vi "MIC communication_MD.vi"() -> ()   [LabVIEW 2012]
uses:
  <vilib>/Utility/VariantDataType/Type.ctl
  GFG/GFGstringGet.vi
  <vilib>/Instr/_visa.llb/VISA Configure Serial Port (Instr).vi
  GFG/GFG library.lvlib
  <vilib>/Utility/VariantDataType/VariantType.lvlib
panel:
  out "read buffer":string
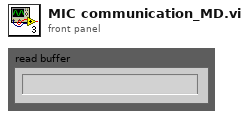
[diagram p1: front panel]
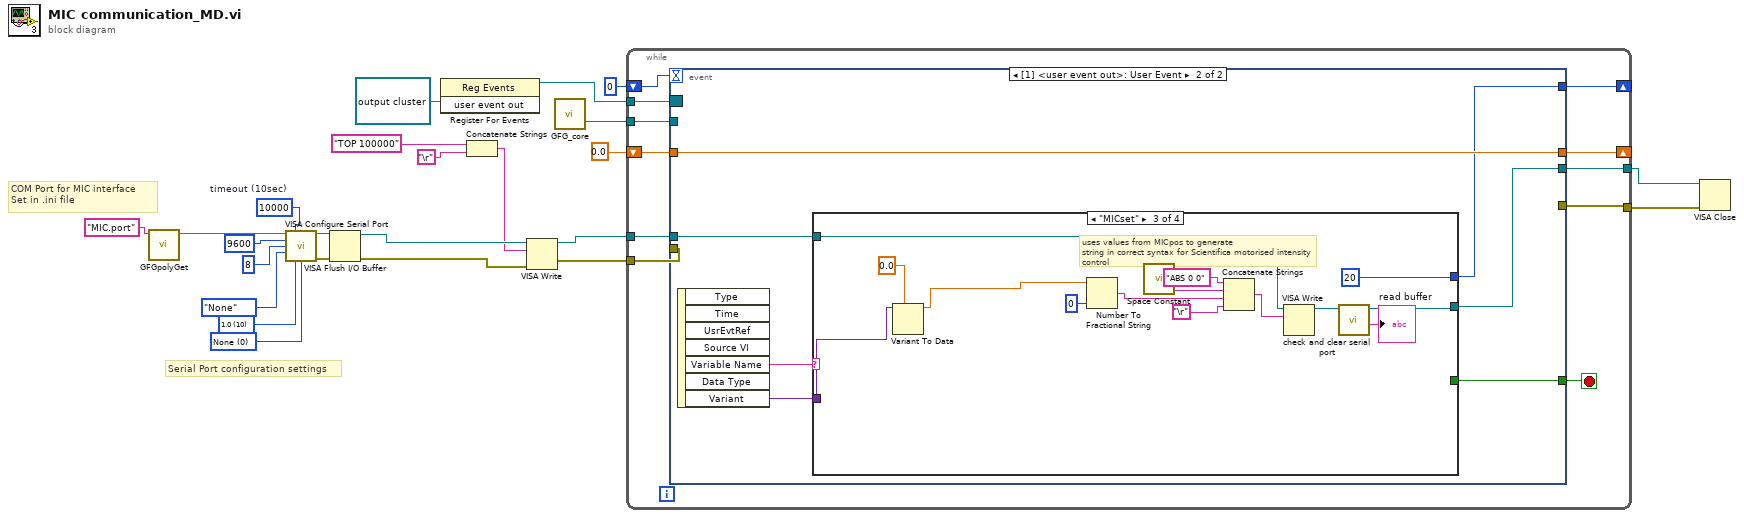
[diagram p0: block diagram]
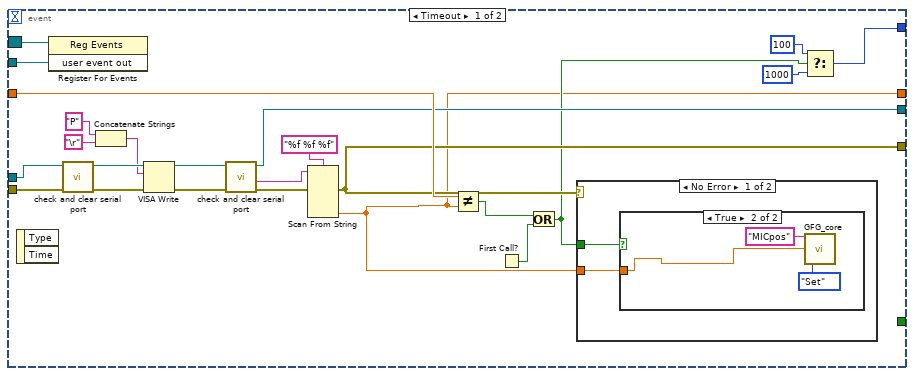
[diagram p2: hidden frame]
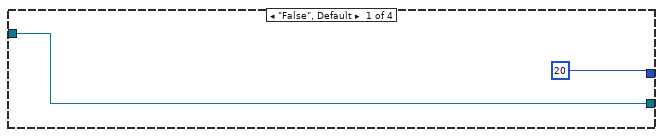
[diagram p5: hidden frame]
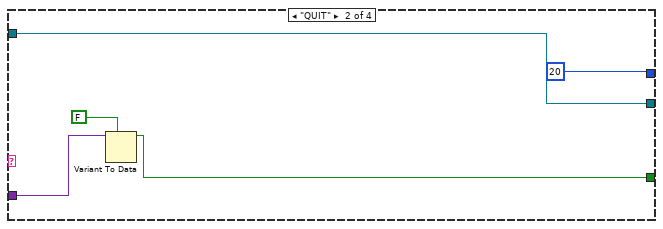
[diagram p6: hidden frame]
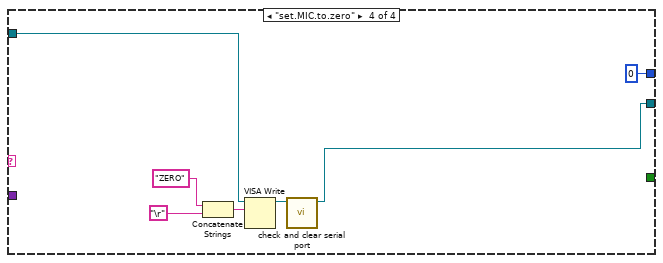
[diagram p7: hidden frame]
diagram:
  w18 = u16 0 items=["None", "XON/XOFF", "RTS/CTS", "XON/XOFF & RTS/CTS", "DTR/DSR", "XON/XOFF & DTR/DSR"] ("flow control (0:none)")
  w19 = u16 10 items=["1.0"=10, "1.5"=15, "2.0"=20] ("stop bits (10: 1 bit)")
  w23 = u32 10000  # timeout (10sec)
  # "COM Port for MIC interface\nSet in .ini file"
  # "Serial Port configuration settings"
  n1 = call-poly "GFGpolyGet.vi"("Variable Name in"="MIC.port") -> ("String"=w15:string)  [unwired: 10 in]
  n2 = call-poly "VISA Configure Serial Port"("VISA resource name"=w15, "timeout (10sec)"=w23, "baud rate (9600)"=u32 9600, "data bits (8)"=u16 8, "parity (0:none)"=enum16{"None", "Odd", "Even", "Mark", "Space"}."None", "stop bits (10: 1 bit)"=w19, "flow control (0:none)"=w18) -> ("VISA resource name out"=w17:refnum<visa-resource-name>, "error out"=w16:errorcluster)  [unwired: 7 in]
  n3 = VISA Flush I/O Buffer(VISA resource name=w17, error in (no error)=w16) -> (VISA resource name out=w7:refnum<visa-resource-name>, error out=w2:errorcluster)  [unwired: 1 in]
  n4 = register-events(refnum<user-event> refnum ("user event out")) -> (reference out=w9:refnum<event-registration>)  [unwired: 2 in, 1 out]
  n5 = Concatenate Strings("TOP 100000" ("write buffer"), "\r") -> (w4:string)
  n6 = VISA Write(VISA resource name=w7, write buffer=w4, error in (no error)=w2) -> (VISA resource name out=w3:refnum<visa-resource-name>, error out=w1:errorcluster)  [unwired: 1 out]
  n7 = call "GFG_core.vi"() -> ("user event out"=w13:refnum<user-event>)  [unwired: 13 in, 6 out]
  n8 = while {
    tunnel: [w35] -> w12
    tunnel: w3 -> [w34]
    shift-right: [w33] -> _
    shift-left: 0.0 -> [w31]
    tunnel: w1 -> [w30]
    tunnel: [w29] -> w11
    shift-right: [w27] -> _
    shift-left: 0 -> [w28]
    tunnel: w13 -> [w26]
    tunnel: w9 -> [w25]
    stop <- w32 stop-if-true
    n9 = event shown="[1] <user event out>: User Event" {
      selector: w25 -> [w39 _]
      dyn-events: _ -> [_ _]
      timeout: w28 -> [_ _]
      tunnel: [w47 w67] -> w35
      tunnel: w34 -> [w56 w68]
      tunnel: [w36 w66] -> w33
      tunnel: [_ w69] -> w32
      tunnel: w31 -> [w59 w66]
      tunnel: w30 -> [w54 _]
      tunnel: [w58 _] -> w29
      tunnel: [w42 w65] -> w27
      tunnel: w26 -> [w38 _]
      event Timeout {
        n10 = event-data() -> ()  [unwired: 1 in, 2 out]
        n11 = register-events(reference=w39, w38) -> ()  [unwired: 1 in, 2 out]
        n12 = call "check and clear serial port.vi"("error in (no error)"=w54, "VISA resource name in"=w56) -> ("error out"=w53:errorcluster, "VISA resource name out"=w55:refnum<visa-resource-name>)  [unwired: 6 in, 2 out]
        n13 = Concatenate Strings("P" ("write buffer"), "\r") -> (w45:string)
        n14 = VISA Write(VISA resource name=w55, write buffer=w45, error in (no error)=w53) -> (VISA resource name out=w49:refnum<visa-resource-name>, error out=w50:errorcluster)  [unwired: 1 out]
        n15 = call "check and clear serial port.vi"("error in (no error)"=w50, "VISA resource name in"=w49) -> ("error out"=w48:errorcluster, "read buffer"=w46:string, "VISA resource name out"=w47:refnum<visa-resource-name>)  [unwired: 6 in, 1 out]
        n16 = Scan From String(format string="%f %f %f", input string=w46, error in=w48) -> (error out=w58:errorcluster, output 3=w36:dbl)  [unwired: 6 in, 2 out]
        n17 = Not Equal?(x=w59, y=w36) -> (x != y?=w37:bool)
        n18 = First Call?() -> (First Call?: T/F=w41:bool)
        n19 = Or(x=w37, y=w41) -> (x .or. y?=w40:bool)
        n20 = case shown="No Error" w58 {
          tunnel: w36 -> [w61 _]
          tunnel: w40 -> [w60 _]
          frame No Error {
            n21 = case shown="True" w60 {
              tunnel: w61 -> [_ w62]
              frame False {
              }
              frame True {
                n22 = call "GFG_core.vi"("Variable Name in"="MICpos", "Variant in"=w62, "Action"=enum16{"Init", "Set", "Get"}."Set") -> ()  [unwired: 10 in, 7 out]
              }
            }
          }
          frame Error {
          }
        }
        n23 = Select(t=100, s=w40, f=1000) -> (s? t:f=w42:i32)
      }
      event User Event {
        n24 = event-data() -> ("Variable Name"=w71:string, "Variant"=w70:variant)  [unwired: 1 in, 5 out]
        n25 = case shown="\"MICset\"" w71 {
          tunnel: [_ w76 _ _] -> w69
          tunnel: w70 -> [_ w78 w84 _]
          tunnel: w68 -> [w73 w75 w89 w95]
          tunnel: [w73 w75 w87 w94] -> w67
          tunnel: [20 20 20 0] -> w65
          frame "False", Default {
          }
          frame "QUIT" {
            n26 = Variant To Data(type=FALSE ("NewVal"), Variant=w78) -> (data=w76:bool)  [unwired: 1 in, 1 out]
          }
          frame "MICset" {
            # "uses values from MICpos to generate\nstring in correct syntax for Scientifica motorised intensity control"
            n27 = Variant To Data(type=0.0 ("moveZabs"), Variant=w84) -> (data=w81:dbl)  [unwired: 1 in, 1 out]
            n28 = Number To Fractional String(number=w81, precision (6)=i16 0) -> (F-format string=w92:string)  [unwired: 2 in]
            n29 = call <vilib>:"Space Constant.vi"() -> ("String"=w91:string)
            n30 = Concatenate Strings("ABS 0 0" ("string"), w91, w92, "\r") -> (w86:string)
            n31 = VISA Write(VISA resource name=w89, write buffer=w86) -> (VISA resource name out=w88:refnum<visa-resource-name>)  [unwired: 1 in, 2 out]
            n32 = call "check and clear serial port.vi"("VISA resource name in"=w88) -> ("read buffer"=→"read buffer":string, "VISA resource name out"=w87:refnum<visa-resource-name>)  [unwired: 7 in, 2 out]
          }
          frame "set.MIC.to.zero" {
            n33 = Concatenate Strings("ZERO" ("write buffer"), "\r") -> (w96:string)
            n34 = VISA Write(VISA resource name=w95, write buffer=w96) -> (VISA resource name out=w97:refnum<visa-resource-name>)  [unwired: 1 in, 2 out]
            n35 = call "check and clear serial port.vi"("VISA resource name in"=w97) -> ("VISA resource name out"=w94:refnum<visa-resource-name>)  [unwired: 7 in, 3 out]
          }
        }
      }
    }
  }
  n36 = VISA Close(VISA resource name=w12, error in (no error)=w11) -> ()  [unwired: 1 out]
